vi "Error Event.vi"(8 "error in (no error)":errorcluster, 11 "Broadcast Actor In":refnum<class "Broadcast Actor.lvclass">) -> (0 "error out":errorcluster)   [LabVIEW 2017, in "Broadcast Actor.lvlib" / "Broadcast Actor.lvclass"]
uses:
  Broadcast Actor.lvclass
  Broadcast Actor.lvclass/Broadcast Actor.ctl
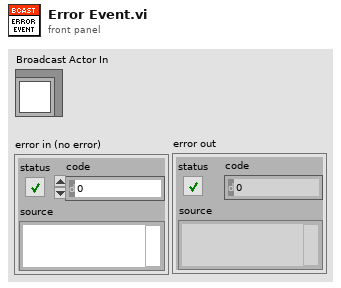
[diagram p1: front panel]
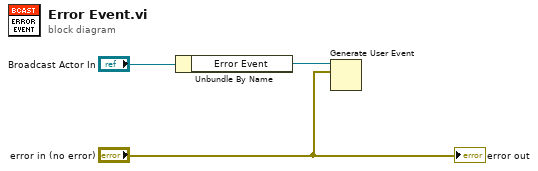
[diagram p0: block diagram]
diagram:
  n1 = Unbundle By Name("Broadcast Actor In") -> ("Error Event"=w2:refnum<user-event>)
  n2 = Generate User Event(user event=w2, event data cluster="error in (no error)") -> ()  [unwired: 2 in, 2 out]
  "error out" <- "error in (no error)"
